vi "F Dwf Digital In Trigger Count Set.vi"(8 "error in (no error)":errorcluster, 9 "fRestart":i32, 10 "cCount":i32, 11 "hdwf":i32) -> (0 "error out":errorcluster, 3 "function return":i32)   [LabVIEW 2021, in "Olasdwf.lvlib"]
doc: "DWFAPI int FDwfDigitalInTriggerCountSet(HDWF hdwf, int cCount, int fRestart);"
uses:
  Olasdwf.lvlib
  Windows/System32/dwf.dll
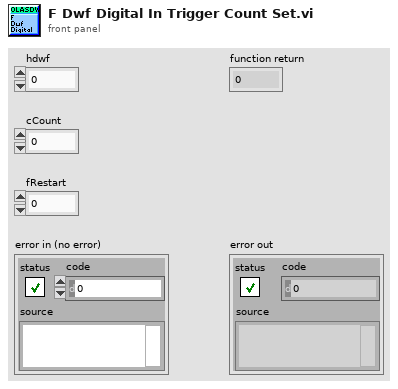
[diagram p1: front panel]
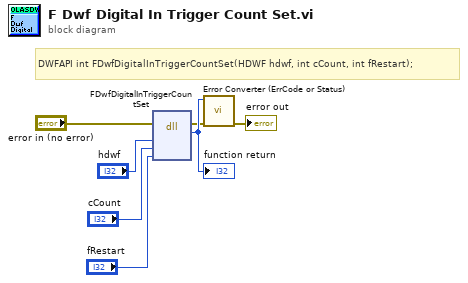
[diagram p0: block diagram]
diagram:
  # "DWFAPI int FDwfDigitalInTriggerCountSet(HDWF hdwf, int cCount, int fRestart);"
  n1 = dll-call lib="/Windows/System32/dwf.*" fn="FDwfDigitalInTriggerCountSet"(error in="error in (no error)", "hdwf"="hdwf", "cCount"="cCount", "fRestart"="fRestart") -> (error out=w2:errorcluster, w7:i32)  [unwired: 5 in, 1 out]
  "function return" <- w7
  n2 = call "Error Converter (ErrCode or Status).vi"("error in (no error)"=w2, "error code"=w7) -> ("error out"=→"error out":errorcluster)  [unwired: 9 in]
